vi "Save Instrument Names.vi"(8 "error in (no error)":errorcluster, 11 "Test Framework in":refnum<class "Test Framework.lvclass">) -> (0 "error out":errorcluster, 3 "Test Framework out":refnum<class "Test Framework.lvclass">)   [LabVIEW 2020, in "Test Framework.lvclass"]
uses:
  Test Framework.lvclass
  Test Framework.lvclass/Test Framework.ctl
  <vilib>/Utility/xml.llb/Write to XML File(string).vi
  Instruments/Instrument.lvclass
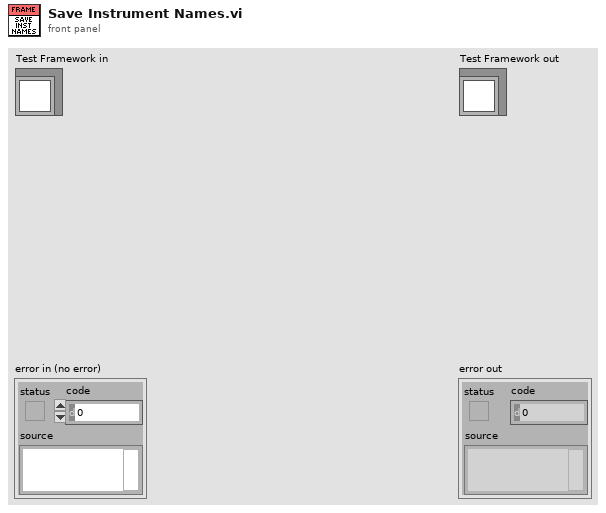
[diagram p1: front panel]
types:
  T1 = cluster{"Instrument Name":string, "Instrument.lvclass":refnum<class "Instrument.lvclass">, "Reference":bool}[]
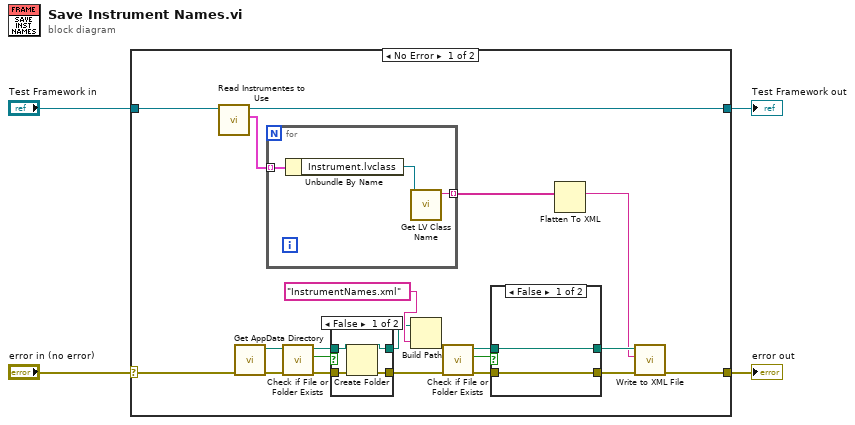
[diagram p0: block diagram]
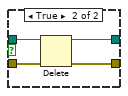
[diagram p3: hidden frame]
diagram:
  n1 = case shown="No Error" "error in (no error)" {
    selector: "error in (no error)" -> [w22 w42]
    tunnel: [w6 w42] -> w3
    tunnel: [w24 w41] -> w1
    tunnel: "Test Framework in" -> [w25 w41]
    frame No Error {
      n2 = call "Read Instrumentes to Use.vi"("Test Framework in"=w25) -> ("Instrumentes to Use"=w23:T1, "Test Framework out"=w24:refnum<class "Test Framework.lvclass">)  [unwired: 9 in]
      n3 = call "Get AppData Directory.vi"("Error In"=w22) -> ("Error Out"=w15:errorcluster, "Folder path"=w14:path)  [unwired: 8 in, 1 out]
      n4 = for {
        tunnel: w23 -> [w40] mode=indexing
        tunnel: [w38] -> w16 mode=indexing
        n5 = Unbundle By Name(w40) -> ("Instrument.lvclass"=w39:refnum<class "Instrument.lvclass">)
        n6 = call <vilib>:"Get LV Class Name.vi"("object"=w39) -> ("class name"=w38:string)  [unwired: 9 in, 1 out]
      }
      n7 = call <vilib>:"Check if File or Folder Exists.vi"("error in (no error)"=w15, "path"=w14) -> ("error out"=w12:errorcluster, "file or folder exists?"=w13:bool, "dup path"=w11:path)  [unwired: 7 in]
      n8 = case shown="False" w13 {
        tunnel: w12 -> [w27 w30]
        tunnel: w11 -> [w28 w31]
        tunnel: [w26 w31] -> w10
        tunnel: [w29 w30] -> w9
        frame False {
          n9 = Create Folder(path (use dialog)=w28, error in=w27) -> (created path=w26:path, error out=w29:errorcluster)  [unwired: 1 in, 1 out]
        }
        frame True {
        }
      }
      n10 = Build Path(base path=w10, name or relative path="InstrumentNames.xml") -> (appended path=w20:path)
      n11 = call <vilib>:"Check if File or Folder Exists.vi"("error in (no error)"=w9, "path"=w20) -> ("error out"=w18:errorcluster, "file or folder exists?"=w19:bool, "dup path"=w17:path)  [unwired: 7 in]
      n12 = case shown="False" w19 {
        tunnel: w18 -> [w33 w37]
        tunnel: w17 -> [w32 w36]
        tunnel: [w33 w35] -> w7
        tunnel: [w32 w34] -> w8
        frame False {
        }
        frame True {
          n13 = Delete(path (use dialog)=w36, error in=w37) -> (deleted path=w34:path, error out=w35:errorcluster)  [unwired: 3 in, 1 out]
        }
      }
      n14 = Flatten To XML(6:w16) -> (2:w5:string)
      n15 = call-poly <vilib>:"Write to XML File.vi"("error in (no error)"=w7, "XML Input"=w5, "XML File Path"=w8) -> ("error out"=w6:errorcluster)  [unwired: 6 in, 2 out]
    }
    frame Error {
    }
  }
  "error out" <- w3
  "Test Framework out" <- w1
